vi "img_read_file_header.vi"(8 "error in":errorcluster, 9 "sector size (512)":u32=512, 11 "hFile":i64) -> (0 "error out":errorcluster, 1 "lpNumberOfBytesRead":u32, 2 "Image Parameters":T1, 3 "hFile out":i64)   [LabVIEW 2015]
doc: "This VI read header information from a file and returns the image properties. The header is one disk sector in size (usually 512 bytes). Each field is 4 bytes:\n\n1) X resolution\n2) Y resolution\n3) Image type\n4) Image border size\n5) Linewidth (pixels)\n6) Bytes per pixel"
uses:
  kernel32.dll
panel:
  in  "cluster":T1
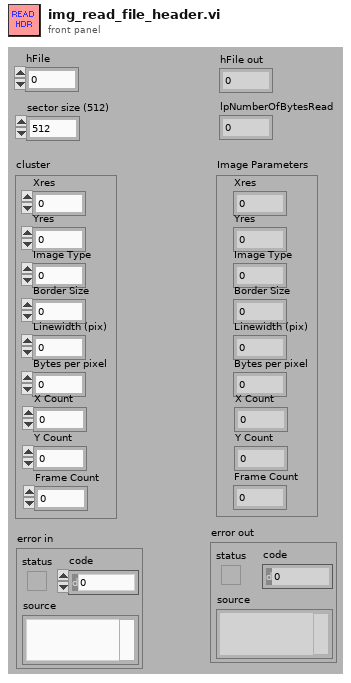
[diagram p1: front panel]
types:
  T1 = cluster{"Xres":u32, "Yres":u32, "Image Type":u32, "Border Size":u32, "Linewidth (pix)":u32, "Bytes per pixel":u32, "X Count":u32, "Y Count":u32, "Frame Count":u32}
  T2 = cluster{"Xres":u32, "Yres":u32, "Image Type":u32, "Border Size":u32, "Linewidth (pix)":u32, "Bytes per pixel":u32, "X Count":u32, "Y Count":u32, "Y Count 2":u32}
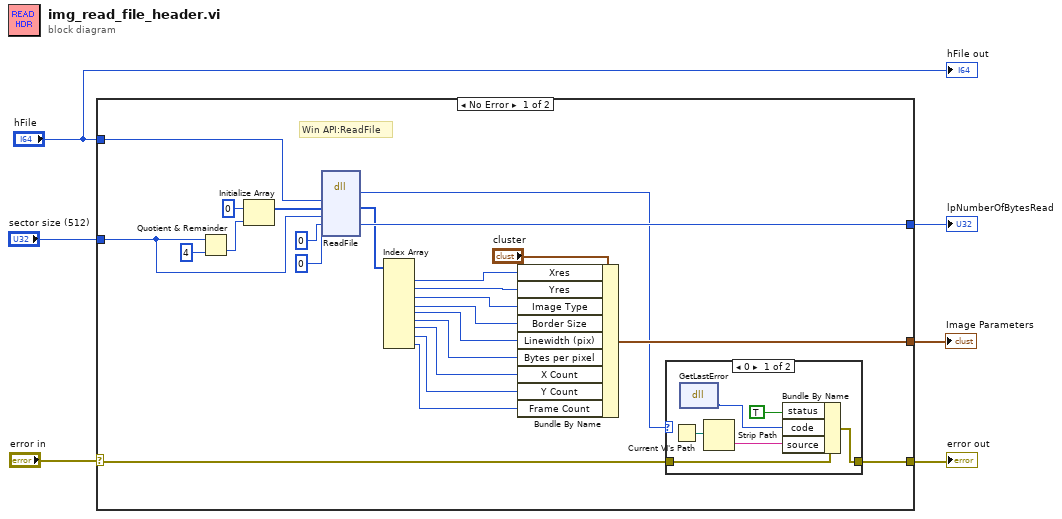
[diagram p0: block diagram]
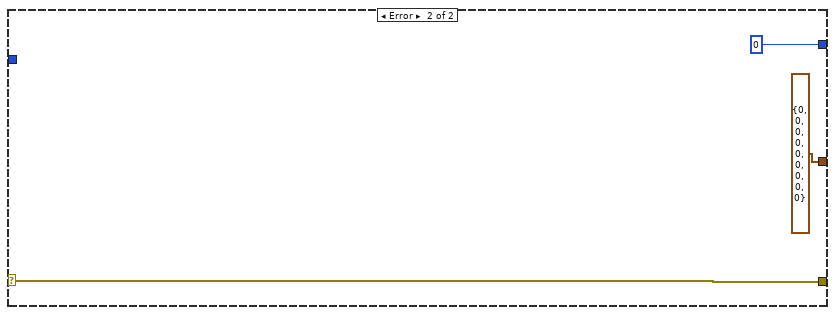
[diagram p3: hidden frame]
diagram:
  n1 = case shown="No Error" "error in" {
    selector: "error in" -> [w13 w40]
    tunnel: "hFile" -> [w30 _]
    tunnel: [w26 u32 0 ("lpNumberOfBytesWritten")] -> w5
    tunnel: [w12 w40] -> w3
    tunnel: [w18 T2 {"Xres"=0, "Yres"=0, "Image Type"=0, "Border Size"=0, "Linewidth (pix)"=0, "Bytes per pixel"=0, "X Count"=0, "Y Count"=0, "Y Count 2"=0} ("cluster")] -> w1
    tunnel: "sector size (512)" -> [w10 _]
    frame No Error {
      # "Win API:ReadFile"
      n2 = Quotient & Remainder(x=w10, y=u32 4 ("element")) -> (floor(x/y)=w15:u32)  [unwired: 1 out]
      n3 = Initialize Array(u32 0 ("element"), w15) -> (w28:u32[])
      n4 = dll-call lib="kernel32.dll" fn="ReadFile"("hFile"=w30, "lpBuffer"=w28, "nNumberOfBytesToRead"=w10, "lpNumberOfBytesRead"=u32 0 ("lpOverlapped"), "lpOverlapped"=u32 0) -> ("error"=w11:i32, "lpBuffer"=w14:u32[], "lpNumberOfBytesRead"=w26:u32)  [unwired: 6 in, 2 out]
      n5 = Index Array(array=w14) -> (element #1=w24:u32, element #2=w23:u32, element #3=w22:u32, element #4=w21:u32, element #5=w20:u32, element #6=w19:u32, element #7=w9:u32, element #8=w8:u32, element #9=w7:u32)  [unwired: 9 in]
      n6 = Bundle By Name(cluster="cluster", "Xres"=w24, "Yres"=w23, "Image Type"=w22, "Border Size"=w21, "Linewidth (pix)"=w20, "Bytes per pixel"=w19, "X Count"=w9, "Y Count"=w8, "Frame Count"=w7) -> (w18:T1)
      n7 = case shown="0" w11 {
        tunnel: w13 -> [w36 w37]
        tunnel: [w35 w37] -> w12
        frame 0 {
          n8 = Current VI's Path() -> (path=w33:path)
          n9 = dll-call lib="kernel32.dll" fn="GetLastError"() -> ("error"=w31:u32)  [unwired: 3 in, 2 out]
          n10 = Strip Path(path=w33) -> (name=w32:string)  [unwired: 1 out]
          n11 = Bundle By Name(cluster=w36, "status"=TRUE, "code"=w31, "source"=w32) -> (w35:errorcluster)
        }
        frame 1, Default {
        }
      }
    }
    frame Error {
    }
  }
  "lpNumberOfBytesRead" <- w5
  "error out" <- w3
  "Image Parameters" <- w1
  "hFile out" <- "hFile"
